vi "SFC_Check Ship.vi"(7 "UserNo":string, 8 "error in (no error)":errorcluster caption="错误输入（无错误）", 9 "DateCode":string, 10 "CartonID":string, 11 "Traceability 引用句柄":refnum<k24>) -> (0 "error out":errorcluster caption="错误输出", 2 "SFC_CheckShipFIFO":string, 3 "Traceability 引用句柄输出":refnum<k24>)   [LabVIEW 2014, in "Traceability.lvlib"]
uses:
  D:/webservice/Traceability.dll
  Traceability.dll
  Traceability.lvlib
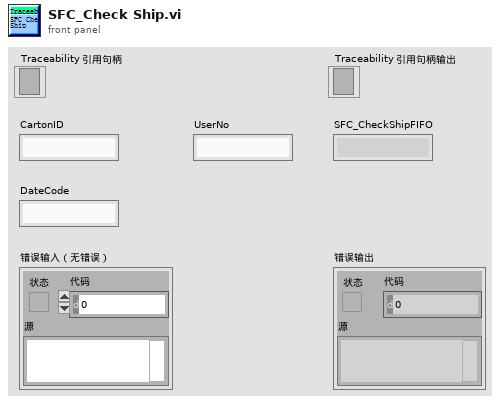
[diagram p1: front panel]
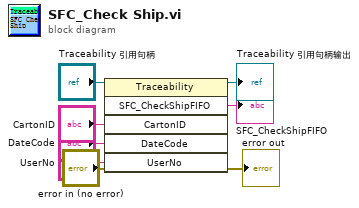
[diagram p0: block diagram]
diagram:
  n1 = invoke class="Traceability" method="SFC_CheckShipFIFO"(reference="Traceability 引用句柄", error in="error in (no error)", "CartonID"="CartonID", "DateCode"="DateCode", "UserNo"="UserNo") -> (reference out=→"Traceability 引用句柄输出":refnum<k24>, error out=→"error out":errorcluster, "SFC_CheckShipFIFO"=→"SFC_CheckShipFIFO":string)  [unwired: 1 in, 3 out]
